vi "Construct Monitor.vi"(7 "error in (no error)":errorcluster, 8 "Enable Logging?":bool, 9 "Monitor Parameters":T2={"channel #"=0, "channel handle"=0, "InstrumentHandle_board"=0, "InstrumentHandle_port"=0, "Queue ID"=0, "channel settings"={"Monitor Settings"={"DefaultCronoMode"=0, "GlbMonBufferSizeIn"=0}, "Rx Board"=0, "Rx Port"=0}, "current log file name"=path "", "monitor queue settings"={"TriggerPosition"=0, "CaptureMode"=0, "Strobe"=0, "MaxFileSize MB (1)"=1}, "Log File Directory"="", "Base name"="", "Timestamp"=FALSE, "log thresholds"={"Segmentation Threshold"=0.0, "Disk Space Percentage"=0.0, "Check Disk Space"=FALSE, "Segment File"=FALSE, "Segment Files By"=0}} {"log thresholds"."Segment Files By" items=["Time", "Size"]; "monitor queue settings"."Strobe" items=["FDX_MON_STROBE_DIS", "FDX_MON_STROBE_STOP", "FDX_MON_STROBE_START"]; "monitor queue settings"."CaptureMode" items=["FDX_MON_SINGLE ", "FDX_MON_CONTINUOUS", "FDX_MON_SELECTIVE", "FDX_MON_RECORDING", "FDX_MON_REROS", "FDX_MON_HMU"]; "channel settings"."Monitor Settings"."DefaultCronoMode" items=["FDX_RX_DEFAULT_ENA_CNT", "FDX_RX_DEFAULT_MON_ENA_ALL", "FDX_RX_DEFAULT_MON_ENA_GOOD"]}, 10 "custom device ref in":T1=18446744073709551615 format="%.0x") -> (0 "error out":errorcluster, 2 "Monitor Execution Unit out":refnum<class "Monitor Execution Unit.lvclass">, 3 "custom device ref out":T1=18446744073709551615 format="%.0x")   [LabVIEW 2020, in "AIM ARINC 664 Engine.lvlib" / "Implementation.lvlib" / "Monitor Execution Unit.lvclass"]
uses:
  Monitor Execution Unit.lvclass
  Execution Unit Factory/Execution Unit Factory.lvclass
  Execution Unit/Execution Unit.lvclass
  Program Files/National Instruments/LabVIEW 2025/instr.lib/AIM GmbH/_AIM 664/_controls/session_monitor_config.ctl
  Program Files/National Instruments/LabVIEW 2025/instr.lib/AIM GmbH/_AIM 664/AIM664LV.lvlib
  Shared/channel_settings_rx.ctl
  Shared/hardware_channels_rx.ctl
  Shared/monitor_queue_settings.ctl
  <vilib>/NI VeriStand/Custom Device API/Custom Device Item Ref.ctl
  <vilib>/NI VeriStand/Custom Device API/Custom Device API.lvlib
  Shared/loggingThreshold_types.ctl
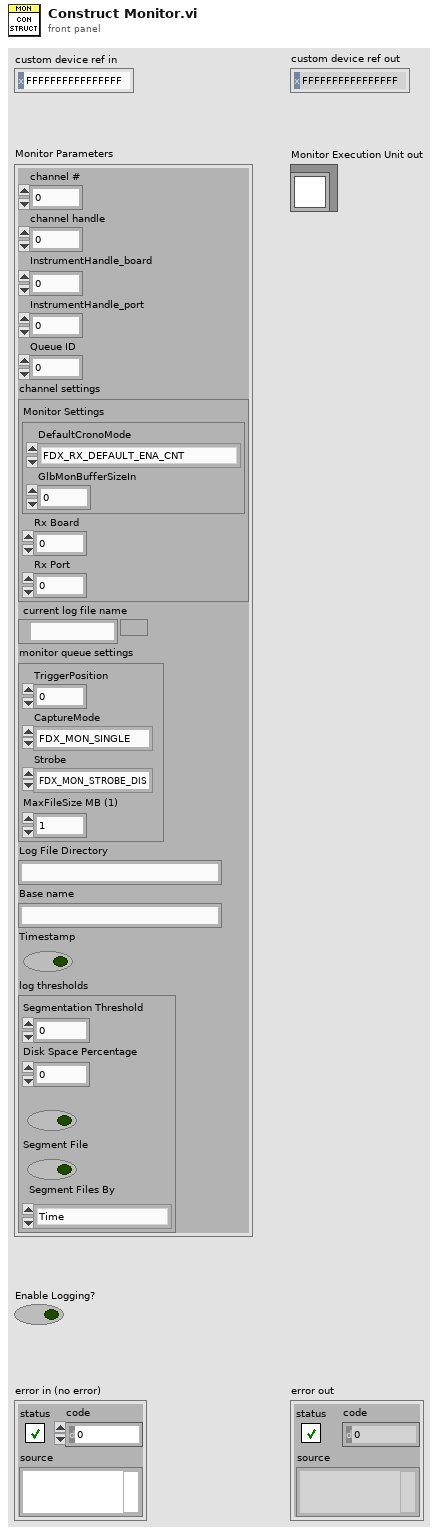
[diagram p1: front panel]
types:
  T1 = typedef "Custom Device API.lvlib/Custom Device Item Ref.ctl" = u64
  T2 = typedef "hardware_channels_rx.ctl" = cluster{"channel #":u16, "channel handle":u64, "InstrumentHandle_board":u32, "InstrumentHandle_port":u32, "Queue ID":u32, "channel settings":T3, "current log file name":path, "monitor queue settings":T5, "Log File Directory":string, "Base name":string, "Timestamp":bool, "log thresholds":T6}
  T3 = typedef "channel_settings_rx.ctl" = cluster{"Monitor Settings":T4, "Rx Board":u32, "Rx Port":u32}
  T4 = typedef "AIM664LV.lvlib/session_monitor_config.ctl" = cluster{"DefaultCronoMode":u32, "GlbMonBufferSizeIn":u32}
  T5 = typedef "monitor_queue_settings.ctl" = cluster{"TriggerPosition":u32, "CaptureMode":u32, "Strobe":u32, "MaxFileSize MB (1)":u32}
  T6 = typedef "loggingThreshold_types.ctl" = cluster{"Segmentation Threshold":dbl, "Disk Space Percentage":dbl, "Check Disk Space":bool, "Segment File":bool, "Segment Files By":u16}
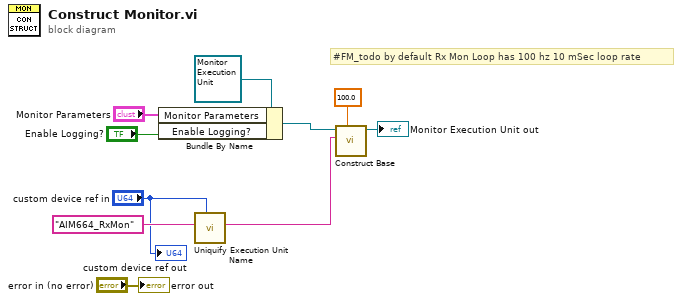
[diagram p0: block diagram]
diagram:
  # "#FM_todo by default Rx Mon Loop has 100 hz 10 mSec loop rate"
  n1 = Bundle By Name(cluster=refnum<class "Monitor Execution Unit.lvclass"> refnum ("Communication Bus Template Interfaces:Implementation.lvlib:Rx Execution Unit.lvclass"), "Monitor Parameters"="Monitor Parameters", "Enable Logging?"="Enable Logging?") -> (w6:refnum<class "Monitor Execution Unit.lvclass">)
  n2 = call "Uniquify Execution Unit Name.vi"("custom device ref"="custom device ref in", "execution unit name"="AIM664_RxMon") -> ("execution unit name out"=w4:string)  [unwired: 9 in]
  n3 = call "Construct Base.vi"("Execution Unit Implementation (default object)"=w6, "identifier"=w4, "async loop rate hz"=100.0) -> ("Execution Unit Out"=→"Monitor Execution Unit out":refnum<class "Monitor Execution Unit.lvclass">)  [unwired: 6 in, 1 out]
  "error out" <- "error in (no error)"
  "custom device ref out" <- "custom device ref in"
